vi "List Packages.vi"(8 "error in (no error)":errorcluster, 11 "Artifactory.VIPM in":refnum<class "Artifactory.VIPM.lvclass">) -> (0 "error out":errorcluster, 1 "found":bool, 2 "VI Packages":string[](array[string]), 3 "Artifactory.VIPM out":refnum<class "Artifactory.VIPM.lvclass">)   [LabVIEW 2021, in "Artifactory.VIPM.lvclass"]
uses:
  Artifactory.VIPM.lvclass
  C:/Repositories/LVOS/Artifactory/lv-src/Artifactory/Artifactory.lvclass
  Artifactory.VIPM.lvclass/Artifactory.VIPM.ctl
  Artifactory/Artifactory.lvclass
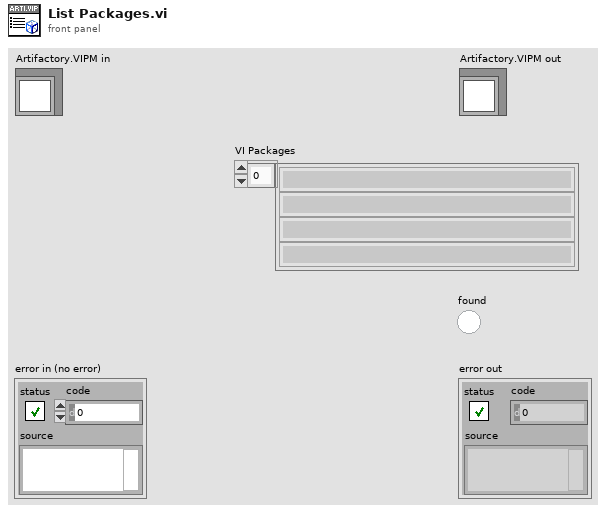
[diagram p1: front panel]
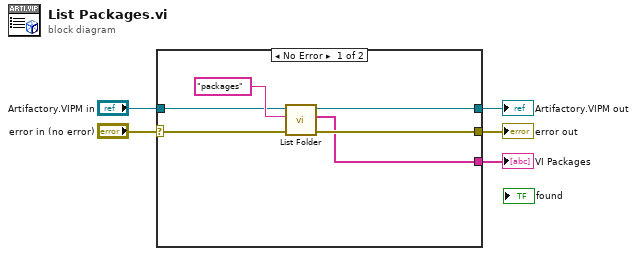
[diagram p0: block diagram]
diagram:
  n1 = case shown="No Error" "error in (no error)" {
    selector: "error in (no error)" -> [w8 w13]
    tunnel: [w7 w13] -> w4
    tunnel: [w10 w12] -> w2
    tunnel: "Artifactory.VIPM in" -> [w9 w12]
    tunnel: [w6 _] -> w1
    frame No Error {
      n2 = call "List Folder.vi"("error in (no error)"=w8, "folder (root)"="packages" ("$Path or Item Name"), "Artifactory in"=w9) -> ("error out"=w7:errorcluster, "Folders"=w6:string[], "Artifactory out"=w10:refnum<class "Artifactory.VIPM.lvclass">)  [unwired: 5 in, 1 out]
    }
    frame Error {
    }
  }
  "error out" <- w4
  "Artifactory.VIPM out" <- w2
  "VI Packages" <- w1
